vi "FormatCANPayload.vi"(4 "ByteFormat":T1, 6 "DataFormat":T2, 11 "Value":sgl) -> (3 "payload":u8[](array[numeric]))   [LabVIEW 2016, in "DSI-RT.lvlib"]
uses:
  DSI-RT.lvlib
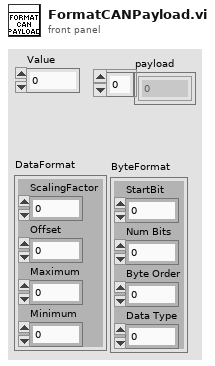
[diagram p1: front panel]
types:
  T1 = cluster{"StartBit":u8, "Num Bits":u8, "Byte Order":u8, "Data Type":u8}
  T2 = cluster{"ScalingFactor":sgl, "Offset":sgl, "Maximum":sgl, "Minimum":sgl}
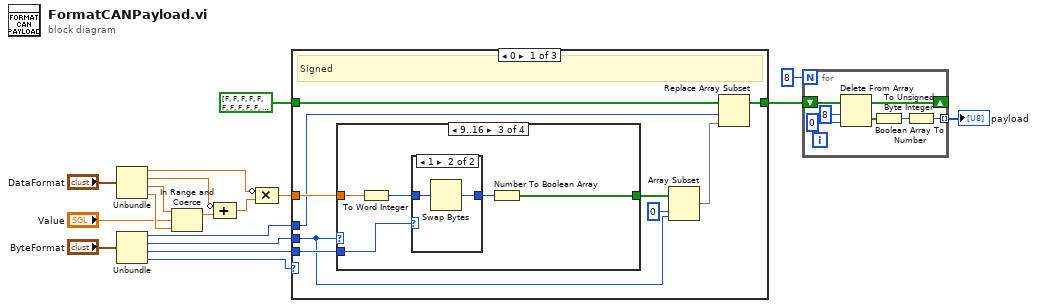
[diagram p0: block diagram]
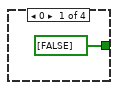
[diagram p2: hidden frame]
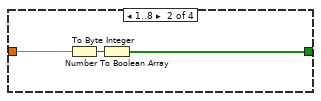
[diagram p3: hidden frame]
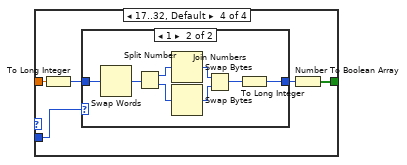
[diagram p5: hidden frame]
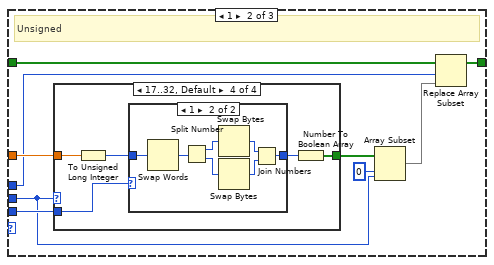
[diagram p7: hidden frame]
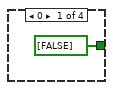
[diagram p8: hidden frame]
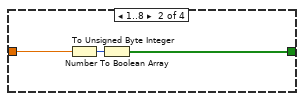
[diagram p9: hidden frame]
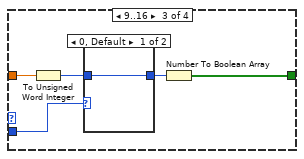
[diagram p10: hidden frame]
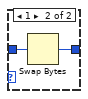
[diagram p11: hidden frame]
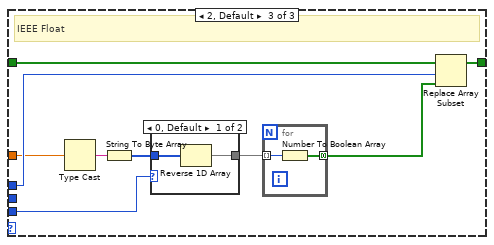
[diagram p13: hidden frame]
diagram:
  n1 = Unbundle("DataFormat") -> ("ScalingFactor"=w10:sgl, "Offset"=w12:sgl, "Maximum"=w16:sgl, "Minimum"=w15:sgl)
  n2 = Unbundle("ByteFormat") -> ("StartBit"=w7:u8, "Num Bits"=w8:u8, "Byte Order"=w5:u8, "Data Type"=w1:u8)
  n3 = In Range and Coerce(upper limit=w16, x="Value", lower limit=w15) -> (coerced(x)=w13:sgl)  [unwired: 1 out]
  n4 = Compound Arithmetic op=ADD(invert w12, w13) -> (w11:sgl)
  n5 = Compound Arithmetic op=MULTIPLY(invert w10, w11) -> (w9:sgl)
  n6 = case shown="0" w1 {
    tunnel: w9 -> [w27 w62 w92]
    tunnel: w8 -> [w19 w55 _]
    tunnel: w7 -> [w25 w60 w95]
    tunnel: bool[] [FALSE, FALSE, FALSE, FALSE, FALSE, FALSE, FALSE, FALSE, FALSE, FALSE, FALSE, FALSE, FALSE, FALSE, FALSE, FALSE, FALSE, FALSE, FALSE, FALSE, FALSE, FALSE, FALSE, FALSE, FALSE, FALSE, FALSE, FALSE, FALSE, FALSE, FALSE, FALSE, FALSE, FALSE, FALSE, FALSE, FALSE, FALSE, FALSE, FALSE, FALSE, FALSE, FALSE, FALSE, FALSE, FALSE, FALSE, FALSE, FALSE, FALSE, FALSE, FALSE, FALSE, FALSE, FALSE, FALSE, FALSE, FALSE, FALSE, FALSE, FALSE, FALSE, FALSE, FALSE] ("payload") -> [w26 w61 w96]
    tunnel: [w24 w59 w94] -> w4
    tunnel: w5 -> [w23 w58 w89]
    frame 0 {
      # "Signed"
      n7 = case shown="9..16" w19 {
        tunnel: w27 -> [_ w31 w36 w44]
        tunnel: [bool[] [FALSE] ("Boolean array") w29 w33 w40] -> w21
        tunnel: w23 -> [_ _ w32 w41]
        frame 0 {
        }
        frame 1..8 {
          n8 = To Byte Integer(number=w31) -> (8bit integer=w30:i8)
          n9 = Number To Boolean Array(number=w30) -> (Boolean array=w29:bool[])
        }
        frame 9..16 {
          n10 = To Word Integer(number=w36) -> (16bit integer=w35:i16)
          n11 = case shown="1" w32 {
            tunnel: w35 -> [w37 w39]
            tunnel: [w37 w38] -> w34
            frame 0, Default {
            }
            frame 1 {
              n12 = Swap Bytes(anything=w39) -> (byte swapped=w38:i16)
            }
          }
          n13 = Number To Boolean Array(number=w34) -> (Boolean array=w33:bool[])
        }
        frame 17..32, Default {
          n14 = To Long Integer(number=w44) -> (32bit integer=w43:i32)
          n15 = case shown="1" w41 {
            tunnel: w43 -> [w45 w53]
            tunnel: [w45 w46] -> w42
            frame 0, Default {
            }
            frame 1 {
              n16 = Swap Words(1:w53) -> (0:w52:i32)
              n17 = Split Number(x=w52) -> (hi(x)=w51:u16, lo(x)=w50:u16)
              n18 = Swap Bytes(anything=w51) -> (byte swapped=w48:u16)
              n19 = Swap Bytes(anything=w50) -> (byte swapped=w49:u16)
              n20 = Join Numbers(hi=w48, lo=w49) -> ((hi.lo)=w47:u32)
              n21 = To Long Integer(number=w47) -> (32bit integer=w46:i32)
            }
          }
          n22 = Number To Boolean Array(number=w42) -> (Boolean array=w40:bool[])
        }
      }
      n23 = Array Subset(array=w21, index=0, length=w19) -> (w20:bool[])
      n24 = Replace Array Subset(array=w26, new element=w20, index=w25) -> (w24:bool[])
    }
    frame 1 {
      # "Unsigned"
      n25 = case shown="17..32, Default" w55 {
        tunnel: w62 -> [_ w66 w71 w79]
        tunnel: [bool[] [FALSE] ("Boolean array") w64 w67 w75] -> w56
        tunnel: w58 -> [_ _ w70 w78]
        frame 0 {
        }
        frame 1..8 {
          n26 = To Unsigned Byte Integer(number=w66) -> (unsigned 8bit integer=w65:u8)
          n27 = Number To Boolean Array(number=w65) -> (Boolean array=w64:bool[])
        }
        frame 9..16 {
          n28 = To Unsigned Word Integer(number=w71) -> (unsigned 16bit integer=w69:u16)
          n29 = case shown="0, Default" w70 {
            tunnel: w69 -> [w72 w74]
            tunnel: [w72 w73] -> w68
            frame 0, Default {
            }
            frame 1 {
              n30 = Swap Bytes(anything=w74) -> (byte swapped=w73:u16)
            }
          }
          n31 = Number To Boolean Array(number=w68) -> (Boolean array=w67:bool[])
        }
        frame 17..32, Default {
          n32 = To Unsigned Long Integer(number=w79) -> (unsigned 32bit integer=w77:u32)
          n33 = case shown="1" w78 {
            tunnel: w77 -> [w80 w87]
            tunnel: [w80 w81] -> w76
            frame 0, Default {
            }
            frame 1 {
              n34 = Swap Words(1:w87) -> (0:w86:u32)
              n35 = Split Number(x=w86) -> (hi(x)=w85:u16, lo(x)=w84:u16)
              n36 = Swap Bytes(anything=w85) -> (byte swapped=w82:u16)
              n37 = Swap Bytes(anything=w84) -> (byte swapped=w83:u16)
              n38 = Join Numbers(hi=w82, lo=w83) -> ((hi.lo)=w81:u32)
            }
          }
          n39 = Number To Boolean Array(number=w76) -> (Boolean array=w75:bool[])
        }
      }
      n40 = Array Subset(array=w56, index=0, length=w55) -> (w54:bool[])
      n41 = Replace Array Subset(array=w61, new element=w54, index=w60) -> (w59:bool[])
    }
    frame 2, Default {
      # "IEEE Float"
      n42 = Type Cast(x=w92) -> (*(type *) &x=w91:string)  [unwired: 1 in]
      n43 = String To Byte Array(string=w91) -> (unsigned byte array=w90:u8[])
      n44 = case shown="0, Default" w89 {
        tunnel: w90 -> [w100 w101]
        tunnel: [w99 w101] -> w88
        frame 0, Default {
          n45 = Reverse 1D Array(array=w100) -> (reversed array=w99:u8[])
        }
        frame 1 {
        }
      }
      n46 = for {
        tunnel: [w98] -> w93 mode=concatenating
        tunnel: w88 -> [w97] mode=indexing
        n47 = Number To Boolean Array(number=w97) -> (Boolean array=w98:bool[])
      }
      n48 = Replace Array Subset(array=w96, new element=w93, index=w95) -> (w94:bool[])
    }
  }
  n49 = for {
    N: 8 -> [_]
    shift-right: [w107] -> _
    shift-left: w4 -> [w108]
    tunnel: [w103] -> w3 mode=indexing
    n50 = Delete From Array(array=w108, length=8, index=0) -> (deleted portion=w105:bool[], array with subset deleted=w107:bool[])
    n51 = Boolean Array To Number(Boolean array=w105) -> (number=w104:u32)
    n52 = To Unsigned Byte Integer(number=w104) -> (unsigned 8bit integer=w103:u8)
  }
  "payload" <- w3
